vi "Convert Error Cluster to Table.vi"(11 "Error Codes":cluster{i32, string}[](array[cluster])=[{8000, "Automotive Diagnostic Command Set: The selected arbitration ID is already in the list of filtered arbitration IDs."}, {8001, "Automotive Diagnostic Command Set: A read buffer in the driver or the software overflowed and surplus data may have been dropped. Other high-priority tasks might be using excessive system resources."}, {-8000, "Automotive Diagnostic Command Set: The handle passed to the function is not valid."}, {-8001, "Automotive Diagnostic Command Set: The selected CAN interface is already active using different settings."}, {-8002, "Automotive Diagnostic Command Set: Diagnostic protocol timeout. A response from the ECU was not received."}, {-8003, "Automotive Diagnostic Command Set: The arbitration ID passed to the function is not valid."}, {-8004, "Automotive Diagnostic Command Set: An internal timeout occurred."}, {-8005, "Automotive Diagnostic Command Set: A required hardware driver support library could not be loaded. Verify that the requested driver is installed or refer to product documentation about specifying the correct driver."}, {-8006, "Automotive Diagnostic Command Set: The name of the interface is not valid."}, {-8007, "Automotive Diagnostic Command Set: The function called is not supported."}, {-8008, "Automotive Diagnostic Command Set: A parameter passed to the function is not valid."}, {-8009, "Automotive Diagnostic Command Set: The selected property is not defined."}, {-8010, "Automotive Diagnostic Command Set: The selected property is read only."}, {-8011, "Automotive Diagnostic Command Set: A callback function has already been defined. To define another callback function, clear the active callback first."}, {-8012, "Automotive Diagnostic Command Set: The function called is not implemented in the nibci.dll. Please update the nibci.dll to a newer version."}, {-8013, "Automotive Diagnostic Command Set: The supplied FPGA bit file is missing one or more mandatory interface elements. Please make sure that your FPGA logic implements the required bridge functionality."}, {-8014, "Automotive Diagnostic Command Set: The selected FPGA bit file was not found. Ensure it is present in the specified directory on the RT target and that you are using the correct path delimiter for the target's operating system."}, {-8017, "Automotive Diagnostic Command Set: The diagnostic service is unknown to the ECU."}, {-8018, "Automotive Diagnostic Command Set: The subfunction of the diagnostic service is unknown to the ECU (invalid format)."}, {-8019, "Automotive Diagnostic Command Set: The length of the request message or the format of the parameters does not match the prescribed requirements for the requested service."}, {-8020, "Automotive Diagnostic Command Set: The response message is too long to be transported via the network."}, {-8033, "Automotive Diagnostic Command Set: The diagnostic service could temporarily not be executed due to other activities (repeat request)."}, {-8034, "Automotive Diagnostic Command Set: The diagnostic service could not be executed due to incorrect conditions (request sequence error)."}, {-8035, "Automotive Diagnostic Command Set: The diagnostic service could not be executed because another function is active (routine not complete)."}, {-8036, "Automotive Diagnostic Command Set: The requested service is out-of-sequence. The ECU expects a different order of the requests issued."}, {-8037, "Automotive Diagnostic Command Set: A gateway reports that a subnet component did not respond."}, {-8038, "Automotive Diagnostic Command Set: A DTC is preventing the service from being executed in the ECU."}, {-8049, "Automotive Diagnostic Command Set: Parameter range error in diagnostic service request."}, {-8051, "Automotive Diagnostic Command Set: The diagnostic service could not be executed due to insufficient security privileges (security access denied)."}, {-8053, "Automotive Diagnostic Command Set: An invalid security key was specified to the ECU."}, {-8054, "Automotive Diagnostic Command Set: The diagnostic service was attempted too often (exceeds number of attempts)."}, {-8055, "Automotive Diagnostic Command Set: The diagnostic service was attempted too quickly (required time delay not expired)."}, {-8112, "Automotive Diagnostic Command Set: Upload/download to the ECU is prevented by a fault condition in the ECU."}, {-8113, "Automotive Diagnostic Command Set: The data transfer operation was aborted due to a fault condition in the ECU."}, {-8114, "Automotive Diagnostic Command Set: The ECU detected an error while erasing or programming its memory (general programming failure)."}, {-8115, "Automotive Diagnostic Command Set: The ECU detected an error in the sequence of block sequence counter values during data transfer."}, {-8126, "Automotive Diagnostic Command Set: The subfunction of the diagnostic service is not supported in the active diagnostic session."}, {-8127, "Automotive Diagnostic Command Set: The diagnostic service is not supported in the active diagnostic session."}, {-8128, "Automotive Diagnostic Command Set: The ECU returned manufacturer specific error code 128."}, {-8129, "Automotive Diagnostic Command Set: The ECU returned manufacturer specific error code 129."}, {-8130, "Automotive Diagnostic Command Set: The ECU returned manufacturer specific error code 130."}, {-8131, "Automotive Diagnostic Command Set: The ECU returned manufacturer specific error code 131."}, {-8132, "Automotive Diagnostic Command Set: The ECU returned manufacturer specific error code 132."}, {-8133, "Automotive Diagnostic Command Set: The ECU returned manufacturer specific error code 133."}, {-8134, "Automotive Diagnostic Command Set: The ECU returned manufacturer specific error code 134."}, {-8135, "Automotive Diagnostic Command Set: The ECU returned manufacturer specific error code 135."}, {-8136, "Automotive Diagnostic Command Set: The ECU returned manufacturer specific error code 136."}, {-8137, "Automotive Diagnostic Command Set: The ECU returned manufacturer specific error code 137."}, {-8138, "Automotive Diagnostic Command Set: The ECU returned manufacturer specific error code 138."}, {-8139, "Automotive Diagnostic Command Set: The ECU returned manufacturer specific error code 139."}, {-8140, "Automotive Diagnostic Command Set: The ECU returned manufacturer specific error code 140."}, {-8141, "Automotive Diagnostic Command Set: The ECU returned manufacturer specific error code 141."}, {-8142, "Automotive Diagnostic Command Set: The ECU returned manufacturer specific error code 142."}, {-8143, "Automotive Diagnostic Command Set: The ECU returned manufacturer specific error code 143."}, {-8144, "Automotive Diagnostic Command Set: The ECU returned manufacturer specific error code 144."}, {-8145, "Automotive Diagnostic Command Set: The ECU returned manufacturer specific error code 145."}, {-8146, "Automotive Diagnostic Command Set: The ECU returned manufacturer specific error code 146."}, {-8147, "Automotive Diagnostic Command Set: The ECU returned manufacturer specific error code 147."}, {-8148, "Automotive Diagnostic Command Set: The ECU returned manufacturer specific error code 148."}, {-8149, "Automotive Diagnostic Command Set: The ECU returned manufacturer specific error code 149."}, {-8150, "Automotive Diagnostic Command Set: The ECU returned manufacturer specific error code 150."}, {-8256, "Automotive Diagnostic Command Set: Invalid frame received by transport layer."}, {-8257, "Automotive Diagnostic Command Set: Out-of-sequence frame received by transport layer."}, {-8258, "Automotive Diagnostic Command Set: Transmit aborted by transport layer due to overflow in the receiver."}, {-8259, "Automotive Diagnostic Command Set: Transmit aborted by transport layer (maximum wait frames received)."}, {-8260, "Automotive Diagnostic Command Set: Diagnostic command timeout. A response from the ECU was not received."}, {-8261, "Automotive Diagnostic Command Set: ISO TP: timeout receiving a Consecutive Frame."}, {-8262, "Automotive Diagnostic Command Set: ISO TP: timeout receiving a Flow Control Frame."}, {-8263, "Automotive Diagnostic Command Set: Transport protocol read timeout. A response from the ECU was not received."}, {-8264, "Automotive Diagnostic Command Set: VW TP 2.0 Protocol error. The selected application type is not supported by the ECU."}, {-8265, "Automotive Diagnostic Command Set: VW TP 2.0 Protocol error. The selected application type is temporarily not supported by the ECU."}, {-8266, "Automotive Diagnostic Command Set: VW TP 2.0 Protocol error. There are temporarily no resources available on the ECU."}, {-8267, "Automotive Diagnostic Command Set: VW TP 2.0 Protocol error. An invalid response was received from the ECU."}, {-8268, "Automotive Diagnostic Command Set: VW TP 2.0 not initialized. Call 'VWTP TP-Request.vi' before calling this VI."}, {-8269, "Automotive Diagnostic Command Set: Receive aborted with OVERLOAD frame due to user settings."}, {-8270, "Automotive Diagnostic Command Set: Invalid response message received."}, {-8300, "Automotive Diagnostic Command Set: DoIP (Diagnostic on Internet Protocol): Transmitted message truncated."}, {-8301, "Automotive Diagnostic Command Set: DoIP (Diagnostic on Internet Protocol): Incorrect target address received."}, {-8302, "Automotive Diagnostic Command Set: DoIP (Diagnostic on Internet Protocol): Incorrect source address received."}, {-8306, "Automotive Diagnostic Command Set: DoIP (Diagnostic on Internet Protocol): Generic header error received."}, {-8344, "Automotive Diagnostic Command Set: DoIP (Diagnostic on Internet Protocol): Routing activation response: Routing activation denied due to unsupported routing activation type."}, {-8345, "Automotive Diagnostic Command Set: DoIP (Diagnostic on Internet Protocol): Routing activation response: Routing activation denied due to confirmation rejected."}, {-8346, "Automotive Diagnostic Command Set: DoIP (Diagnostic on Internet Protocol): Routing activation response: Routing activation denied due to missing authentication."}, {-8347, "Automotive Diagnostic Command Set: DoIP (Diagnostic on Internet Protocol): Routing activation response: Routing activation denied because the SA is already registered and active on a different TCP_DATA socket."}, {-8348, "Automotive Diagnostic Command Set: DoIP (Diagnostic on Internet Protocol): Routing activation response: Routing activation denied because an SA different from the table connection entry was received on the already activated TCP_DATA socket."}, {-8349, "Automotive Diagnostic Command Set: DoIP (Diagnostic on Internet Protocol): Routing activation response: Routing activation denied because all concurrently supported TCP_DATA sockets are registered and active."}, {-8350, "Automotive Diagnostic Command Set: DoIP (Diagnostic on Internet Protocol): Routing activation response: Routing activation denied due to unknown source address."}, {-8352, "Automotive Diagnostic Command Set: DoIP (Diagnostic on Internet Protocol): Routing activation response: OEM specific message 254."}, {-8353, "Automotive Diagnostic Command Set: DoIP (Diagnostic on Internet Protocol): Routing activation response: OEM specific message 253."}, {-8354, "Automotive Diagnostic Command Set: DoIP (Diagnostic on Internet Protocol): Routing activation response: OEM specific message 252."}, {-8355, "Automotive Diagnostic Command Set: DoIP (Diagnostic on Internet Protocol): Routing activation response: OEM specific message 251."}, {-8356, "Automotive Diagnostic Command Set: DoIP (Diagnostic on Internet Protocol): Routing activation response: OEM specific message 250."}, {-8357, "Automotive Diagnostic Command Set: DoIP (Diagnostic on Internet Protocol): Routing activation response: OEM specific message 249."}, {-8358, "Automotive Diagnostic Command Set: DoIP (Diagnostic on Internet Protocol): Routing activation response: OEM specific message 248."}, {-8359, "Automotive Diagnostic Command Set: DoIP (Diagnostic on Internet Protocol): Routing activation response: OEM specific message 247."}, {-8360, "Automotive Diagnostic Command Set: DoIP (Diagnostic on Internet Protocol): Routing activation response: OEM specific message 246."}, {-8361, "Automotive Diagnostic Command Set: DoIP (Diagnostic on Internet Protocol): Routing activation response: OEM specific message 245."}, {-8362, "Automotive Diagnostic Command Set: DoIP (Diagnostic on Internet Protocol): Routing activation response: OEM specific message 244."}, {-8363, "Automotive Diagnostic Command Set: DoIP (Diagnostic on Internet Protocol): Routing activation response: OEM specific message 243."}, {-8364, "Automotive Diagnostic Command Set: DoIP (Diagnostic on Internet Protocol): Routing activation response: OEM specific message 242."}, {-8365, "Automotive Diagnostic Command Set: DoIP (Diagnostic on Internet Protocol): Routing activation response: OEM specific message 241."}, {-8366, "Automotive Diagnostic Command Set: DoIP (Diagnostic on Internet Protocol): Routing activation response: OEM specific message 240."}, {-8367, "Automotive Diagnostic Command Set: DoIP (Diagnostic on Internet Protocol): Routing activation response: OEM specific message 239."}, {-8368, "Automotive Diagnostic Command Set: DoIP (Diagnostic on Internet Protocol): Routing activation response: OEM specific message 238."}, {-8369, "Automotive Diagnostic Command Set: DoIP (Diagnostic on Internet Protocol): Routing activation response: OEM specific message 237."}, {-8370, "Automotive Diagnostic Command Set: DoIP (Diagnostic on Internet Protocol): Routing activation response: OEM specific message 236."}, {-8371, "Automotive Diagnostic Command Set: DoIP (Diagnostic on Internet Protocol): Routing activation response: OEM specific message 235."}, {-8372, "Automotive Diagnostic Command Set: DoIP (Diagnostic on Internet Protocol): Routing activation response: OEM specific message 234."}, {-8373, "Automotive Diagnostic Command Set: DoIP (Diagnostic on Internet Protocol): Routing activation response: OEM specific message 233."}, {-8374, "Automotive Diagnostic Command Set: DoIP (Diagnostic on Internet Protocol): Routing activation response: OEM specific message 232."}, {-8375, "Automotive Diagnostic Command Set: DoIP (Diagnostic on Internet Protocol): Routing activation response: OEM specific message 231."}, {-8376, "Automotive Diagnostic Command Set: DoIP (Diagnostic on Internet Protocol): Routing activation response: OEM specific message 230."}, {-8377, "Automotive Diagnostic Command Set: DoIP (Diagnostic on Internet Protocol): Routing activation response: OEM specific message 229."}, {-8378, "Automotive Diagnostic Command Set: DoIP (Diagnostic on Internet Protocol): Routing activation response: OEM specific message 228."}, {-8379, "Automotive Diagnostic Command Set: DoIP (Diagnostic on Internet Protocol): Routing activation response: OEM specific message 227."}, {-8380, "Automotive Diagnostic Command Set: DoIP (Diagnostic on Internet Protocol): Routing activation response: OEM specific message 226."}, {-8381, "Automotive Diagnostic Command Set: DoIP (Diagnostic on Internet Protocol): Routing activation response: OEM specific message 225."}, {-8382, "Automotive Diagnostic Command Set: DoIP (Diagnostic on Internet Protocol): Routing activation response: OEM specific message 224."}, {-8400, "Automotive Diagnostic Command Set: DoIP (Diagnostic on Internet Protocol): Incorrect diagnostic message response received."}, {-8402, "Automotive Diagnostic Command Set: DoIP (Diagnostic on Internet Protocol): Diagnostic message negative ACK: Invalid source address."}, {-8403, "Automotive Diagnostic Command Set: DoIP (Diagnostic on Internet Protocol): Diagnostic message negative ACK: Unknown target address."}, {-8404, "Automotive Diagnostic Command Set: DoIP (Diagnostic on Internet Protocol): Diagnostic message negative ACK: Diagnostic message too large."}, {-8405, "Automotive Diagnostic Command Set: DoIP (Diagnostic on Internet Protocol): Diagnostic message negative ACK: Out of memory."}, {-8406, "Automotive Diagnostic Command Set: DoIP (Diagnostic on Internet Protocol): Diagnostic message negative ACK: Target unreachable."}, {-8407, "Automotive Diagnostic Command Set: DoIP (Diagnostic on Internet Protocol): Diagnostic message negative ACK: Unknown network."}, {-8408, "Automotive Diagnostic Command Set: DoIP (Diagnostic on Internet Protocol): Diagnostic message negative ACK: Transport protocol error."}, {-8409, "Automotive Diagnostic Command Set: An internal error occurred."}, {-8465, "Automotive Diagnostic Command Set: A third-party CAN driver reported an error. Verify your settings and hardware configuration"}, {-8466, "Automotive Diagnostic Command Set: An unexpected error occurred in the BCI layer."}, {-8467, "Automotive Diagnostic Command Set: The interface device reported a critical error. Data may have been lost or corrupted."}, {8468, "Automotive Diagnostic Command Set: A read buffer in the driver or the software overflowed and surplus data may have been dropped. Other high-priority tasks might be using excessive system resources."}, {-8469, "Automotive Diagnostic Command Set: A write buffer in the driver or the software overflowed and the provided data was not transmitted. Please wait for parts of the buffer to be processed and try again."}, {-8470, "Automotive Diagnostic Command Set: A frame in a format invalid for the current communication mode was received or requested to be transmitted, e.g. the data size was outside of the allowed range."}, {-8471, "Automotive Diagnostic Command Set: ISO CAN FD mode is not supported for the selected interface and its installed driver version. Refer to product documentation for information about hardware and driver version support."}, {-8472, "Automotive Diagnostic Command Set: The driver could not be loaded for the selected NI-CAN device. Verify that the driver is installed or refer to product documentation about specifying the correct driver."}, {-8473, "Automotive Diagnostic Command Set: This error is currently not defined but reserved for future extensions."}, {-8474, "Automotive Diagnostic Command Set: This error is currently not defined but reserved for future extensions."}, {-8475, "Automotive Diagnostic Command Set: This error is currently not defined but reserved for future extensions."}, {-8476, "Automotive Diagnostic Command Set: This error is currently not defined but reserved for future extensions."}, {-8477, "Automotive Diagnostic Command Set: This error is currently not defined but reserved for future extensions."}, {-8478, "Automotive Diagnostic Command Set: This error is currently not defined but reserved for future extensions."}, {-8479, "Automotive Diagnostic Command Set: This error is currently not defined but reserved for future extensions."}, {-8480, "Automotive Diagnostic Command Set: This error is currently not defined but reserved for future extensions."}, {-1074384895, "NI-XNET:  (Hex 0xBFF63001) An internal error occurred in the NI-XNET driver. Solution: Contact National Instruments and provide the log files found in %LOCALAPPDATA%\\National Instruments\\NI-XNET\\log. Note that this location might be hidden on your computer. For LabVIEW RT systems, log files are located in /ni-rt/nixnet/log or /var/lib/ni-xnet/log."}, {-1074384894, "NI-XNET:  (Hex 0xBFF63002) Board self test failed(code 2). Solution: Try reinstalling the driver or switching the slot(s) of the board(s). If the error persists, contact National Instruments."}, {-1074384893, "NI-XNET:  (Hex 0xBFF63003) Board self test failed(code 3). Solution: Try reinstalling the driver or switching the slot(s) of the board(s). If the error persists, contact National Instruments."}, {-1074384892, "NI-XNET:  (Hex 0xBFF63004) Board self test failed(code 4). Solution: Try reinstalling the driver or switching the slot(s) of the board(s). If the error persists, contact National Instruments."}, {-1074384891, "NI-XNET:  (Hex 0xBFF63005) Board self test failed(code 5). Solution: Try reinstalling the driver or switching the slot(s) of the board(s). If the error persists, contact National Instruments."}, {-1074384890, "NI-XNET:  (Hex 0xBFF63006) Board self test failed(code 6). Solution: Try reinstalling the driver or switching the slot(s) of the board(s). If the error persists, contact National Instruments."}, {-1074384889, "NI-XNET:  (Hex 0xBFF63007) Computer went to hibernation mode and the board lost power. Solution: Prevent the computer from going to hibernation mode in the control panel."}, {-1074384888, "NI-XNET:  (Hex 0xBFF63008) A write queue overflowed. Solution: Wait until queue space becomes available and retry."}, {-1074384887, "NI-XNET:  (Hex 0xBFF63009) The board's firmware did not answer a command. Solution: Stop your application and execute a self test. Try deactivating/reactivating the driver in the Device Manager. If the problem persists, contact National Instruments."}, {-1074384886, "NI-XNET:  (Hex 0xBFF6300A) The operation timed out. Solution: Specify a timeout long enough to complete the operation, or change the operation in a way that it can get completed in less time (e.g., read less data)."}, {-1074384885, "NI-XNET:  (Hex 0xBFF6300B) A read queue overflowed. Solution: Reduce your data rate or call Read more frequently."}, {-1074384884, "NI-XNET:  (Hex 0xBFF6300C) The Read buffer is too small to hold a single frame. Solution: Provide a buffer large enough."}, {-1074384883, "NI-XNET:  (Hex 0xBFF6300D) You tried to open the same frame twice. This is not permitted. Solution: Open each frame only once."}, {-1074384882, "NI-XNET:  (Hex 0xBFF6300E) You tried to open the same stream object twice. This is not permitted. Solution: Open each stream object only once."}, {-1074384881, "NI-XNET:  (Hex 0xBFF6300F) Self test is not possible since the board is in use by an application. Solution: Stop all NI-XNET applications before executing a self test."}, {-1074384880, "NI-XNET:  (Hex 0xBFF63010) Allocation of memory failed. You do not have sufficient memory in the LabVIEW target. Solution: Add more RAM or try to use fewer resources in your applications (arrays, XNET sessions, etc)."}, {-1074384879, "NI-XNET:  (Hex 0xBFF63011) The maximum number of sessions was exceeded. Solution: Use fewer sessions."}, {-1074384878, "NI-XNET:  (Hex 0xBFF63012) The maximum number of sessions has been exceeded. Solution: Use fewer sessions."}, {-1074384877, "NI-XNET:  (Hex 0xBFF63013) The maximum number of devices has been detected. Solution: Use fewer devices."}, {-1074384876, "NI-XNET:  (Hex 0xBFF63014) A driver support file is missing. Solution: Try reinstalling the driver. If the error persists, contact National Instruments."}, {-1074384875, "NI-XNET:  (Hex 0xBFF63015) This indicates that a NULL pointer or an empty string was passed to a function. The user should verify that the parameters passed in make sense for the given function."}, {-1074384874, "NI-XNET:  (Hex 0xBFF63016) The maximum number of schedules has been detected. Solution: Use fewer schedules."}, {-1074384873, "NI-XNET:  (Hex 0xBFF63017) Board self test failed (code 17). Solution: Try reinstalling the driver or switching the slot(s) of the board(s). If the error persists, contact National Instruments."}, {-1074384872, "NI-XNET:  (Hex 0xBFF63018) You cannot start an NI-XNET application while a self test is in progress. Solution: Complete the self test before starting any NI-XNET applications."}, {-1074384864, "NI-XNET:  (Hex 0xBFF63020) An invalid reference has been passed to a NI-XNET session function. Solution: Only pass reference retrieved from Create Session, or from an IO name of a session in LabVIEW project."}, {-1074384863, "NI-XNET:  (Hex 0xBFF63021) An invalid reference has been passed to a NI-XNET system function. Solution: Only pass a valid system reference."}, {-1074384862, "NI-XNET:  (Hex 0xBFF63022) A device reference was expected for a NI-XNET session function. Solution: Only pass a device reference."}, {-1074384861, "NI-XNET:  (Hex 0xBFF63023) An interface reference was expected for a NI-XNET session function. Solution: Only pass an interface reference."}, {-1074384860, "NI-XNET:  (Hex 0xBFF63024) You have configured a property that conflicts with the current mode of the session. For example, you have created a CAN output session with a frame configured with a Timing Type = Cyclic and a Transmit Time of 0."}, {-1074384859, "NI-XNET:  (Hex 0xBFF63025) The XNET Create Timing Source VI is supported only on LabVIEW Real-Time targets currently running the Phar Lap ETS Real-Time Operating System."}, {-1074384858, "NI-XNET:  (Hex 0xBFF63026) You tried to create more than one LabVIEW timing source for a single interface. Only one timing source per interface is supported. The timing source remains until the top-level VI is idle (no longer running). Solution: Call the XNET Create Timing Source VI only once per interface. You can use the timing source with multiple timed structures (e.g., timed loops)."}, {-1074384857, "NI-XNET:  (Hex 0xBFF63027) You invoked two or more VIs simultaneously for the same session, and those VIs do not support overlap. For example, you attempted to invoke two Read VIs at the same time for the same session. Solution: Wire the error cluster from one VI to another, to enforce sequential execution for the session."}, {-1074384856, "NI-XNET:  (Hex 0xBFF63028) You are trying to start an interface that is missing bus power for the transceiver. Some physical layers on NI-XNET hardware are internally powered, but others require external power for the port to operate. This error occurs when starting an interface on hardware that requires external power when no power is detected. Solution: Supply proper voltage to your transceiver. Refer to the NI-XNET Hardware Overview in the NI-XNET Hardware and Software Manual for more information."}, {-1074384855, "NI-XNET:  (Hex 0xBFF63029) The connection with a CompactDAQ chassis was lost, and the host software and modules are out of sync.  There is no direct recovery for this problem until the chassis is reset. Solutions: Call DAQmx Reset Device as the first VI or function in your application, prior to creating XNET sessions. Alternately, you could reset the CompactDAQ chassis in Measurement and Automation Explorer (MAX)."}, {-1074384783, "NI-XNET:  (Hex 0xBFF63071) The transceiver value set is invalid (for this port, e.g., LS on a HS port) or you are trying to perform an operation that requires a different transceiver (e.g., trying to change the state of a disconnected transceiver). Solution: Set a valid value."}, {-1074384782, "NI-XNET:  (Hex 0xBFF63072) The baud rate value set is invalid. Solution: Set a valid value."}, {-1074384781, "NI-XNET:  (Hex 0xBFF63073) No baud rate value has been set. Solution: Set a valid value."}, {-1074384780, "NI-XNET:  (Hex 0xBFF63074) The bit timing values set are invalid. Solution: Set valid values."}, {-1074384779, "NI-XNET:  (Hex 0xBFF63075) The baud rate set does not match the transceiver's allowed range. Solution: Change either the baud rate or the transceiver."}, {-1074384778, "NI-XNET:  (Hex 0xBFF63076) The configured terminal is not known for this interface. Solution: Make sure that that you pass in a valid value to Connect Terminals or Disconnect Terminals."}, {-1074384777, "NI-XNET:  (Hex 0xBFF63077) The configured terminal is inappropriate for the hardware. For example, setting a source to FrontPanel0 on XNET hardware that does not have front-panel trigger inputs, or selecting PXI_Clk10 for a non-PXI device. Solution: Pick an appropriate terminal for the hardware."}, {-1074384776, "NI-XNET:  (Hex 0xBFF63078) The source that you connected to the Master Timebase destination is missing. When the start trigger is received, the interface verifies that a signal is present on the configured source. This check has determined that this signal is missing. Solution: Verify that your cables are configured correctly and that your timebase source is generating an appropriate waveform."}, {-1074384775, "NI-XNET:  (Hex 0xBFF63079) The source that you connected to the Master Timebase destination is not generating an appropriate signal. When the start trigger is received, the interface verifies that a signal of a known frequency is present on the configured source. This check has determined that this source is generating a signal, but that the signal is not one of the supported frequencies for this hardware. Solution: Verify that your source is generating a signal at a supported frequency."}, {-1074384774, "NI-XNET:  (Hex 0xBFF6307A) You are trying to disconnect a synchronization terminal that is not currently connected. Solution: Only disconnect synchronization terminals that have previously been connected."}, {-1074384773, "NI-XNET:  (Hex 0xBFF6307B) You are trying to connect a synchronization terminal that is already in use. For example, you are trying to connect a trigger line to the Master Timebase when a different trigger line is already connected to the Master Timebase. Solution: Only connect to synchronization terminals that are not currently in use."}, {-1074384772, "NI-XNET:  (Hex 0xBFF6307C) You are trying to connect an XNET terminal as a source terminal,  but the desired XNET terminal is not valid as a source terminal. Solution: Only connect valid source terminals to the source terminal in XNET Connect Terminals."}, {-1074384771, "NI-XNET:  (Hex 0xBFF6307D) You are trying to connect an XNET terminal as a destination terminal, but the desired XNET terminal is not valid as a destination terminal. Solution: Only connect valid destination terminals to the destination terminal in XNET Connect Terminals."}, {-1074384770, "NI-XNET:  (Hex 0xBFF6307E) You are trying to connect two XNET terminals that are incompatible. Solution: Only connect a source and destination terminals that are compatible with each other."}, {-1074384769, "NI-XNET:  (Hex 0xBFF6307F) The source that you connected to the Master Timebase destination has disappeared. When the start trigger is received, the interface verifies that a signal is present on the configured source. This check has determined that this signal was present, but while the interface was running, the signal disappeared, so all timebase configuration has reverted to using the onboard (unsynchronized) oscillator. Solution: Verify that your cables are configured correctly and that your timebase source is generating an appropriate waveform the entire time your application is running."}, {-1074384768, "NI-XNET:  (Hex 0xBFF63080) You called Read (State : FlexRay : Cycle Macrotick), and the FlexRay Macrotick is not connected as the master timebase of the interface. Solution: Call Connect Terminals to connect source of FlexRay Macrotick to destination of Master Timebase."}, {-1074384767, "NI-XNET:  (Hex 0xBFF63081) The database specified could not be opened. Solution: Check that the alias and/or the file exists and that it is a valid database. Also, make sure the path does not contain Unicode characters, which cannot be utilized by NI-XNET."}, {-1074384766, "NI-XNET:  (Hex 0xBFF63082) The cluster was not found in the database. Solution: Make sure you only initialize a cluster in a session that is defined in the database."}, {-1074384765, "NI-XNET:  (Hex 0xBFF63083) The frame was not found in the database. Solution: Make sure you only initialize frames in a session that are defined in the database."}, {-1074384764, "NI-XNET:  (Hex 0xBFF63084) The signal was not found in the database. Solution: Make sure you only initialize signals in a session that are defined in the database."}, {-1074384763, "NI-XNET:  (Hex 0xBFF63085) A necessary property for a cluster was not found in the database. Solution: Make sure you only initialize a cluster in a session that is completely defined in the database."}, {-1074384762, "NI-XNET:  (Hex 0xBFF63086) A necessary property for a frame was not found in the database. Solution: Make sure you only initialize frames in a session that are completely defined in the database."}, {-1074384761, "NI-XNET:  (Hex 0xBFF63087) A necessary property for a signal was not found in the database. Solution: Make sure you only initialize signals in a session that are completely defined in the database."}, {-1074384760, "NI-XNET:  (Hex 0xBFF63088) Multiple clusters have been specified in one session, either directly (Stream I/O), or through the signals or frames specified. Solution: Make sure that in one session, you open only one cluster, including frames or signals that belong to the same cluster."}, {-1074384759, "NI-XNET:  (Hex 0xBFF63089) You specified a database of ':subordinate:' for a session mode other than mode of Frame Input Stream. Solution: Either open a Frame Input Stream session, or use a real or in-memory database."}, {-1074384758, "NI-XNET:  (Hex 0xBFF6308A) The interface name given does not specify a valid and existing interface. Solution: Use a valid and existing interface. These can be obtained using MAX, XNET system properties, or the LabVIEW XNET Interface IO name. If you are using CompactRIO, refer to the topic \"Getting Started with CompactRIO\" in the NI-XNET Hardware and Software Help."}, {-1074384757, "NI-XNET:  (Hex 0xBFF6308B) The operation is invalid for this interface (e.g., you tried to open a set of FlexRay frames on a CAN interface, or tried to request a CAN property from a FlexRay interface). Solution: Run this operation on a suitable interface."}, {-1074384756, "NI-XNET:  (Hex 0xBFF6308C) You tried to set the AutoStart property to FALSE for an Input session. This is not allowed. Solution: Do not set the AutoStart property (TRUE is default)."}, {-1074384755, "NI-XNET:  (Hex 0xBFF6308D) The property ID you specified is not valid (or not valid for the current session mode or form factor). Check to make sure the installed XNET driver supports the specified property ID."}, {-1074384754, "NI-XNET:  (Hex 0xBFF6308E) The contents of the property is bigger than the size specified. Use the nxGetPropertySize function to determine the size of the buffer needed."}, {-1074384753, "NI-XNET:  (Hex 0xBFF6308F) The function you called is not defined for the session mode (e.g., you called a frame I/O function on a signal I/O session)."}, {-1074384752, "NI-XNET:  (Hex 0xBFF63090) The data that you passed to XNET Write or XNET Read is too small to hold all the data specified for the session. Solution: Determine the number of elements (frames or signals) that you configured for the session, and pass that number of elements to XNET Write or XNET Read."}, {-1074384751, "NI-XNET:  (Hex 0xBFF63091) For Signal Output sessions, the multiplexer signals used in the session must be specified explicitly in the signal list."}, {-1074384750, "NI-XNET:  (Hex 0xBFF63092) You used an XNET Session IO name, and that session was not found in your LabVIEW project. Solution: Within LabVIEW project, right-click the target (RT or My Computer), and select New > NI-XNET Session. Add the VI that uses the session under the target. If you are using the session with a built application (.EXE), ensure that you copy the built configuration file nixnetSession.txt such that it resides in the same folder as the executable."}, {-1074384749, "NI-XNET:  (Hex 0xBFF63093) You used the same XNET session name in multiple top-level VIs, which is not supported. Solution: Use each session in only one top-level VI (application) at a time."}, {-1074384748, "NI-XNET:  (Hex 0xBFF63094) To execute this function properly, the session's list must contain only one frame. Solution: Break your session up into multiple, each of which contains only one frame."}, {-1074384747, "NI-XNET:  (Hex 0xBFF63095) You used the same alias for different database files which is not allowed. Solution: Use each alias only for a single database file."}, {-1074384746, "NI-XNET:  (Hex 0xBFF63096) You try to deploy a database file while another deployment is in progress. Solution: Wait until the other deployment has finished and try again."}, {-1074384745, "NI-XNET:  (Hex 0xBFF63097) A signal or frame session has been opened, but it does not contain signals or frames. Solution: Specify at least one signal or frame."}, {-1074384744, "NI-XNET:  (Hex 0xBFF63098) The session mode selected is not supported by the protocol of the specified interface. Solution: Choose a valid session mode."}, {-1074384743, "NI-XNET:  (Hex 0xBFF63099) A session was created by references, but no database references have been specified. Solution: Specify at least one appropriate database reference (i.e., signal or frame or cluster ref depending on the session mode)."}, {-1074384742, "NI-XNET:  (Hex 0xBFF6309A) The interface has already been opened with different cluster settings than the ones specified for this session. Solution: Make sure that the cluster settings agree for the interface, or use a different interface."}, {-1074384741, "NI-XNET:  (Hex 0xBFF6309B) The cycle repetition of a frame in the database for the FlexRay protocol is invalid. Solution: Make sure that the cycle repetition is a power of 2 between 1 and 64."}, {-1074384740, "NI-XNET:  (Hex 0xBFF6309C) You called XNET Clear for the session, then tried to perform another operation. Solution: Defer clear (session close) until you are done using it. This error can also occur if you branch a wire after creating the session. Solution: Do not branch a session to multiple flows in the diagram."}, {-1074384739, "NI-XNET:  (Hex 0xBFF6309D) You called Create Session VI with a list of items that does not match the mode. This includes using: 1) signal items for a Frame I/O mode 2) frame items for a Signal I/O mode 3) cluster item for a mode other than Frame Input Stream or Frame Output Stream"}, {-1074384738, "NI-XNET:  (Hex 0xBFF6309E) You tried to create a new session while the interface is already running. Solution: Create all sessions before starting any of them."}, {-1074384737, "NI-XNET:  (Hex 0xBFF6309F) You wrote a frame whose payload length is larger than the maximum payload allowed by the database (e.g., wrote 10 bytes for CAN frame, max 8 bytes). Solution: Never write more payload bytes than the Payload Length Maximum property of the session."}, {-1074384736, "NI-XNET:  (Hex 0xBFF630A0) You called a Read function with a nonzero timeout, and you used a negative numberToRead. Negative value for numberToRead requests all available data from the Read, which is ambiguous when used with a timeout. Solutions: 1) Pass timeout of 0 and numberToRead of -1, to request all available data. 2) Pass timeout > 0, and numberToRead > 0, to wait for a specific number of data elements."}, {-1074384735, "NI-XNET:  (Hex 0xBFF630A1) Timestamps are not (yet) supported for Write Signal XY. Solution: Do not provide a timestamp array for Write Signal XY."}, {-1074384734, "NI-XNET:  (Hex 0xBFF630A2) The condition parameter passed to Wait is not known. Solution: Pass a valid parameter."}, {-1074384733, "NI-XNET:  (Hex 0xBFF630A3) You attempted an I/O operation, but the session is not yet started (and the AutoStart property is set to FALSE). Solution: Call Start before you use this I/O operation."}, {-1074384732, "NI-XNET:  (Hex 0xBFF630A4) The maximum number of Wait operations has been exceeded. Solution: If you are waiting for multiple events on the interface, use fewer Wait operations on this interface (even for multiple sessions). If you are waiting for multiple events for a frame (e.g., transmit complete), use only one Wait at a time for that frame."}, {-1074384731, "NI-XNET:  (Hex 0xBFF630A5) You used an invalid name for an XNET Device. Solution: Get valid XNET Device names from the XNET System properties (only)."}, {-1074384730, "NI-XNET:  (Hex 0xBFF630A6) A terminal name passed to ConnectTerminals or DisconnectTerminals is unknown. Solution: Only pass valid names."}, {-1074384729, "NI-XNET:  (Hex 0xBFF630A7) You tried to blink the port LEDs but these are currently busy. Solution: Stop all applications running on that port; do not access it from MAX or LV Project."}, {-1074384728, "NI-XNET:  (Hex 0xBFF630A8) You tried to set a FlexRay keyslot ID that is not listed as valid in the database. Solution: Only pass slot IDs of frames that have the startup or sync property set in the database."}, {-1074384727, "NI-XNET:  (Hex 0xBFF630A9) You tried to set a queue size that is bigger than the maximum allowed. Solution: Specify an in-range queue size."}, {-1074384726, "NI-XNET:  (Hex 0xBFF630AA) You wrote a frame whose payload length is different than the payload length configured by the database. Solution: Never write a different payload length for a frame that is different than the configured payload length."}, {-1074384725, "NI-XNET:  (Hex 0xBFF630AB) The index to indicate an session list element is too large. Solution: Specify an index in the range 0 ... NumInList-1."}, {-1074384724, "NI-XNET:  (Hex 0xBFF630AC) You have tried to create a session that is invalid for the mode of the driver/firmware. For example, you are using the Replay Exclusive mode for Stream Output and you have an output session open."}, {-1074384723, "NI-XNET:  (Hex 0xBFF630AD) The trigger signal for a frame is allowed only in Single Point Signal sessions (Input or Output). For Output Single Point Signal sessions, only one trigger signal is allowed per frame. Solution: Do not use the trigger signal, or change to a single point I/O session."}, {-1074384722, "NI-XNET:  (Hex 0xBFF630AE) To execute this function properly, the session's list must contain only one cluster. Solution: Use only one cluster in the session."}, {-1074384721, "NI-XNET:  (Hex 0xBFF630AF) You attempted to convert a CAN or LIN frame with a payload length greater than 8. For example, you may be converting a frame that uses a higher layer transport protocol, such as SAE-J1939. NI-XNET currently supports conversion of CAN/LIN frames only (layer 2). Solutions: 1) Implement higher layer protocols (including signal conversion) within your code. 2) Contact National Instruments to request this feature in a future version."}, {-1074384720, "NI-XNET:  (Hex 0xBFF630B0) Allocation of memory failed for the data returned from LabVIEW XNET Read. Solutions: 1) Wire a smaller \"number to read\" to XNET Read (default -1 uses queue size).  2) For Signal Input Waveform, use a smaller resample rate. 3) Set smaller value for session's queue size property (default is large to avoid loss of data)."}, {-1074384719, "NI-XNET:  (Hex 0xBFF630B1) Allocation of memory failed in the firmware. Solutions: 1) Create less firmware objects 2) Set smaller value for output session's queue size property (default is large to avoid loss of data)."}, {-1074384718, "NI-XNET:  (Hex 0xBFF630B2) The NI-XNET driver no longer can communicate with the device. Solution: Make sure the device has not been removed from the computer."}, {-1074384717, "NI-XNET:  (Hex 0xBFF630B3) A LIN schedule has an invalid priority. Solution: Use a valid priority (0 = NULL schedule, 1..254 = Run once schedule, 255 = Continuous schedule)."}, {-1074384716, "NI-XNET:  (Hex 0xBFF630B4) (Dis)ConnectTerminals is not allowed for XNET C Series modules. Solution: To connect the module start trigger, use the Session property Interface Source Terminal Start Trigger."}, {-1074384715, "NI-XNET:  (Hex 0xBFF630B5) You requested a time (like Start or Communication Time) before the event has happened. Solution: Request the time only after it occurred."}, {-1074384714, "NI-XNET:  (Hex 0xBFF630B6) An internal input queue overflowed. Solution: Attempt to pull data from the hardware faster. If you are connected by an external bus (for example, USB or Ethernet), you can try to use a faster connection."}, {-1074384713, "NI-XNET:  (Hex 0xBFF630B7) A bad firmware image file can not be loaded to the hardware. Solution: Uninstall and reinstall the NI-XNET software as the default firmware file may be corrupt. If you are using a custom firmware file, try rebuilding it."}, {-1074384712, "NI-XNET:  (Hex 0xBFF630B8) The encoding of embedded network data (CAN, FlexRay, LIN, etc.) within the TDMS file is invalid. Solutions: 1) In the application that wrote (created) the logfile, and the application in which you are reading it, confirm that both use the same major version for frame data encoding (NI_network_frame_version property of the TDMS channel). 2) Ensure that your file was not corrupted."}, {-1074384711, "NI-XNET:  (Hex 0xBFF630B9) The NI-XNET hardware no longer can communicate with the transceiver cable. This may be due to the cable being removed, a power loss event, an over voltage condition on the power input, or a general communication error. Solution: Make sure the dongle is properly latched and, for some hardware, external power is properly applied. To detect other errors, stop your application and execute a self test."}, {-1074384710, "NI-XNET:  (Hex 0xBFF630BA) The NI-XNET driver timed out when performing low-level communication with the device. This could occur if the device was removed, communication with its parent chassis failed, or a general hardware failure occurred."}, {-1074384709, "NI-XNET:  (Hex 0xBFF630BB) A transfer to the C Series module was aborted. This could occur if the cDAQ chassis was disconnected, reset, power cycled, or another issue occurred that interfered with communication. Solution: Verify that the cDAQ chassis and NI-XNET module are both present, powered, and operational in Measurement and Automation Explorer (MAX). A reset of the cDAQ chassis may be necessary to recover from the error."}, {-1074384708, "NI-XNET:  (Hex 0xBFF630BC) An invalid value has been specified for the CAN FD ISO Mode. Solution: Specify a valid value."}, {-1074384704, "NI-XNET:  (Hex 0xBFF630C0) A property value was out of range or incorrect. Solution: Specify a correct value."}, {-1074384703, "NI-XNET:  (Hex 0xBFF630C1) Integration of the interface into the FlexRay cluster failed, so communication did not start for the interface. Solution: Check the cluster and/or interface parameters and verify that there are startup frames defined."}, {-1074384688, "NI-XNET:  (Hex 0xBFF630D0) The PDU was not found in the database. Solution: Make sure you initialize only PDUs in a session that are defined in the database."}, {-1074384687, "NI-XNET:  (Hex 0xBFF630D1) A necessary property for a PDU was not found in the database. Solution: Make sure you initialize only PDUs in a session that are completely defined in the database."}, {-1074384686, "NI-XNET:  (Hex 0xBFF630D2) You tried to open the same PDU twice. This is not permitted. Solution: Open each PDU only once."}, {-1074384685, "NI-XNET:  (Hex 0xBFF630D3) You can access this database object only by PDU, not by frame. Solution: For CAN and LIN, this is not supported by the current version of NI-XNET; for FlexRay, make sure the database is set to use PDUs."}, {-1074384640, "NI-XNET:  (Hex 0xBFF63100) Remote communication with the LabVIEW RT target failed. Solution: Check if NI-XNET has been installed on the RT target and check if the NI-XNET RPC server has been started."}, {-1074384639, "NI-XNET:  (Hex 0xBFF63101) File transfer communication with the LabVIEW Real-Time (RT) target failed. Solution: Check if the RT target has been powered on, the RT target has been connected to the network, and if the IP address settings are correct. If the RT target is password protected, make sure you provided the correct user credentials."}, {-1074384638, "NI-XNET:  (Hex 0xBFF63102) File transfer to the LabVIEW Real-Time (RT) target failed, because the required files could not be accessed. Solution: You may have executed a VI that opened the database, but did not close. If that is the case, you should change the VI to call Database Close, then reboot the RT controller to continue."}, {-1074384637, "NI-XNET:  (Hex 0xBFF63103) The database file you want to use is already assigned to another alias. Solution: Each database file can only be assigned to a single alias. Use the alias that is already assigned to the database instead."}, {-1074384636, "NI-XNET:  (Hex 0xBFF63104) An internal file used by NI-XNET could not be accessed. Solution: Make sure that the internal NI-XNET files are not write protected and that the directories for these files exist."}, {-1074384635, "NI-XNET:  (Hex 0xBFF63105) The file cannot be deployed because another file deployment is already active. Solution: Wait until the other file deployment has finished, and try again."}, {-1074384617, "NI-XNET:  (Hex 0xBFF63117) The nixnet.dll or one of its components could not be loaded. Solution: Try reinstalling NI-XNET. If the error persists, contact National Instruments."}, {-1074384610, "NI-XNET:  (Hex 0xBFF6311E) You attempted to perform an action on a session or interface that is started, and the action that requires the session/interface to be stopped. Solution: Stop the object before performing this action."}, {-1074384609, "NI-XNET:  (Hex 0xBFF6311F) You have passed a default payload to the firmware where the number of bytes in the payload is larger than the number of bytes that this frame can transmit. Solution: Decrease the number of bytes in your default payload."}, {-1074384605, "NI-XNET:  (Hex 0xBFF63123) You attempted to set a CAN arbitration ID with an invalid value. For example, a CAN standard arbitration ID supports only 11 bits. If you attempt to set a standard arbitration ID that uses more than 11 bits, this error is returned. Solution: Use a valid arbitration ID."}, {-1074384604, "NI-XNET:  (Hex 0xBFF63124) You attempted to set a LIN ID with an invalid value. For example, a LIN ID supports only 6 bits. If you attempt to set an ID that uses more than 6 bits, this error is returned. Solution: Use a valid LIN ID."}, {-1074384592, "NI-XNET:  (Hex 0xBFF63130) Too many open files. NI-XNET allows up to 7 database files to be opened simultaneously. Solution: Open fewer files."}, {-1074384591, "NI-XNET:  (Hex 0xBFF63131) Bad reference has been passed to a database function, e.g., a session reference, or frame reference to retrieve properties from a signal."}, {-1074384590, "NI-XNET:  (Hex 0xBFF63132) Creating a database file failed. Solution: Verify access rights to the destination directory or check if overwritten file has read only permission."}, {-1074384589, "NI-XNET:  (Hex 0xBFF63133) A cluster with the same name already exists in the database. Solution: Use another name for this cluster."}, {-1074384588, "NI-XNET:  (Hex 0xBFF63134) A frame with the same name already exists in the cluster. Solution: Use another name for this frame."}, {-1074384587, "NI-XNET:  (Hex 0xBFF63135) A signal with the same name already exists in the frame. Solution: Use another name for this signal."}, {-1074384586, "NI-XNET:  (Hex 0xBFF63136) An ECU with the same name already exists in the cluster. Solution: Use another name for this ECU."}, {-1074384585, "NI-XNET:  (Hex 0xBFF63137) A subframe with the same name already exists in the frame. Solution: Use another name for this subframe."}, {-1074384584, "NI-XNET:  (Hex 0xBFF63138) The operation is improper for the protocol in use, e.g., you cannot assign FlexRay channels to a CAN frame."}, {-1074384583, "NI-XNET:  (Hex 0xBFF63139) Wrong parent relationship for a child that you are creating with XNET Database Create."}, {-1074384581, "NI-XNET:  (Hex 0xBFF6313B) The retrieved required property is not defined on the specified object. Solution: Make sure that your database file has this property defined or that you set it in the objects created in memory."}, {-1074384580, "NI-XNET:  (Hex 0xBFF6313C) The feature is not supported under LabVIEW RT, e.g.Save Database"}, {-1074384579, "NI-XNET:  (Hex 0xBFF6313D) The object name contains unsupported characters. The name must contain just alphanumeric characters and the underscore, but cannot begin with a digit. The maximum size is 128."}, {-1074384578, "NI-XNET:  (Hex 0xBFF6313E) Unsupported database format. For reading a database, the extension must be .xml, .dbc, .ncd, or .ldf. For saving, the extension must be .xml or .ldf"}, {-1074384577, "NI-XNET:  (Hex 0xBFF6313F) Database object not found (e.g., an object with given name does not exist)."}, {-1074384576, "NI-XNET:  (Hex 0xBFF63140) Database cache file cannot be removed or replaced on the disc (e.g., file is write-protected)."}, {-1074384575, "NI-XNET:  (Hex 0xBFF63141) You are trying to write a read-only property, e.g., the mux value on a signal is a read only property (can be changed on the subframe)."}, {-1074384574, "NI-XNET:  (Hex 0xBFF63142) You are trying to change a signal to be a mux signal, but a mux is already defined in this frame"}, {-1074384572, "NI-XNET:  (Hex 0xBFF63144) You are trying to define FlexRay in-cycle-repetition slots before defining the first slot. Define the first slot (frame ID) before defining in-cycle-repetition slots."}, {-1074384571, "NI-XNET:  (Hex 0xBFF63145) You are trying to define FlexRay in-cycle-repetition channels before defining the first channels. Define the Channel Assignment on a frame before defining in-cycle-repetition channels."}, {-1074384570, "NI-XNET:  (Hex 0xBFF63146) You must define the protocol before setting this property (e.g., the frame ID has a different meaning in a CAN or FlexRay cluster)."}, {-1074384569, "NI-XNET:  (Hex 0xBFF63147) The database information on the real-time system has been created with an older NI-XNET version. This version is no longer supported. To correct this error, re-deploy your database to the real-time system."}, {-1074384568, "NI-XNET:  (Hex 0xBFF63148) Frame ConfigStatus: A signal within the frame exceeds the frame boundaries (Payload Length)."}, {-1074384567, "NI-XNET:  (Hex 0xBFF63149) Frame ConfigStatus: A signal within the frame overlaps another signal."}, {-1074384566, "NI-XNET:  (Hex 0xBFF6314A) Frame ConfigStatus: A integer signal within the frame is defined with more than 52 bits. Not supported."}, {-1074384565, "NI-XNET:  (Hex 0xBFF6314B) Frame ConfigStatus: Frame is defined with an invalid payload size. Allowed sizes vary by bus type and application protocol."}, {-1074384564, "NI-XNET:  (Hex 0xBFF6314C) You are trying to add transmitted FlexRay frames to an ECU, with at least two of them having Startup or Sync property on. Only one Sync or Startup frame is allowed to be sent by an ECU."}, {-1074384563, "NI-XNET:  (Hex 0xBFF6314D) You are trying to add TX/RX frames to an ECU which are defined in a different cluster than the ECU."}, {-1074384562, "NI-XNET:  (Hex 0xBFF6314E) Database name parameter is incorrect. Solution: Use a valid name for the database, e.g., \":memory:\" for in-memory database."}, {-1074384561, "NI-XNET:  (Hex 0xBFF6314F) Database object is locked because it is used in a session. Solution: Configure the database before using it in a session."}, {-1074384560, "NI-XNET:  (Hex 0xBFF63150) Alias name passed to a function is not defined. Solution: Define the alias before calling the function."}, {-1074384559, "NI-XNET:  (Hex 0xBFF63151) Database file cannot be saved because frames are assigned to FlexRay channels not defined in the cluster. Solution: Verify that all frames in the FlexRay cluster are assigned to an existing cluster channel."}, {-1074384558, "NI-XNET:  (Hex 0xBFF63152) Frame ConfigStatus: This FlexRay frame transmitted in a dynamic segment uses both channels A and B. This is not allowed. Solution: Use either channel A or B."}, {-1074384557, "NI-XNET:  (Hex 0xBFF63153) Database is locked because it is being modified by an another instance of the same application. Solution: Close the database in the other application instance."}, {-1074384556, "NI-XNET:  (Hex 0xBFF63154) A frame name is ambiguous (e.g., a frame with the same name exists in another cluster). Solution: Specify the cluster name for the frame using the required syntax."}, {-1074384555, "NI-XNET:  (Hex 0xBFF63155) A signal name is ambiguous (e.g., a signal with the same name exists in another frame). Solution: Use <frame>.<signal> syntax for the signal."}, {-1074384554, "NI-XNET:  (Hex 0xBFF63156) An ECU name is ambiguous (e.g., an ECU with the same name exists in another cluster). Solution: Specify the cluster name for the ECU using the required syntax."}, {-1074384553, "NI-XNET:  (Hex 0xBFF63157) A subframe name is ambiguous (e.g., a subframe with the same name exists in another cluster). Solution: Specify the cluster name for the subframe using the required syntax."}, {-1074384552, "NI-XNET:  (Hex 0xBFF63158) A LIN schedule name is ambiguous (e.g., a schedule with the same name exists in another cluster). Solution: Specify the cluster name for the schedule using the required syntax."}, {-1074384551, "NI-XNET:  (Hex 0xBFF63159) A LIN schedule with the same name already exists in the database. Solution: Use another name for this schedule."}, {-1074384550, "NI-XNET:  (Hex 0xBFF6315A) Multiplexers (mode-dependent signals) are not supported when the given protocol is used. Solution: Contact National Instruments to see whether there is a newer NI-XNET version that supports multiplexers for the given protocol."}, {-1074384549, "NI-XNET:  (Hex 0xBFF6315B) Saving a FIBEX file containing a LIN cluster is not supported in this NI-XNET version. Solution: Contact National Instruments to see whether there is a newer NI-XNET version that supports saving a FIBEX file that contains a LIN cluster."}, {-1074384548, "NI-XNET:  (Hex 0xBFF6315C) This property requires an ECU configured as LIN master to be present in this cluster. Solution: Create a LIN master ECU in this cluster."}, {-1074384547, "NI-XNET:  (Hex 0xBFF6315D) You have tried to create a session using a frame that is incompatible with the selected session type. For example, you are using a LIN diagnostic frame with a single point output session."}, {-1074384546, "NI-XNET:  (Hex 0xBFF6315E) You cannot mix open of NI-XNET database objects as both manual and automatic. You open manually by calling the Database Open VI. You open automatically when you 1) wire the IO name directly to a property node or VI, 2) branch a wire to multiple data flows on the diagram, 3) use the IO name with a VI or property node after closing it with the Database Close VI. Solution: Change your diagram to use the manual technique in all locations (always call Open and Close VIs), or to use the automatic technique in all locations (never call Open or Close VIs)."}, {-1074384545, "NI-XNET:  (Hex 0xBFF6315F) Due to problems in LabVIEW versions 8.5 through 8.6.1, automatic open of NI-XNET database objects is not supported. You open automatically when you 1) wire the IO name directly to a property node or VI, 2) branch a wire to multiple data flows on the diagram, 3) use the IO name with a VI or property node after closing it with the Database Close VI. Solution: Change your diagram to call the Database Open VI prior to any use (VI or property node) in a data flow (including a new wire branch). Change your diagram to call the Database Close VI when you are finished using the database in your application."}, {-1074384544, "NI-XNET:  (Hex 0xBFF63160) You called a Write function with the number of array elements (frames or signals) different than the number of elements configured in the session (such as the \"list\" parameter of the Create Session function). Solution: Write the same number of elements as configured in the session."}, {-1074384543, "NI-XNET:  (Hex 0xBFF63161) You used XNET session from multiple LabVIEW projects (or multiple executables), which NI-XNET does not support. Solution: Run XNET sessions in only one LabVIEW project at a time."}, {-1074384542, "NI-XNET:  (Hex 0xBFF63162) When an XNET session is used at runtime, all sessions in the same scope are created on the interface. The same scope is defined as all sessions within the same LabVIEW project which use the same cluster and interface (same physical cable configuration). If you attempt to use a session in the same scope after 
